vi "initImageAll.vi"() -> (3 "Refnum out":T1)   [LabVIEW 2013, in "MagAnalysis_Online.lvclass"]
uses:
  MagAnalysis_Online.lvclass
  IMAQ Image.ctl
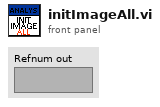
[diagram p1: front panel]
types:
  T1 = typedef "IMAQ Image.ctl" = refnum<image>
  T2 = typedef "Image Type" = u32
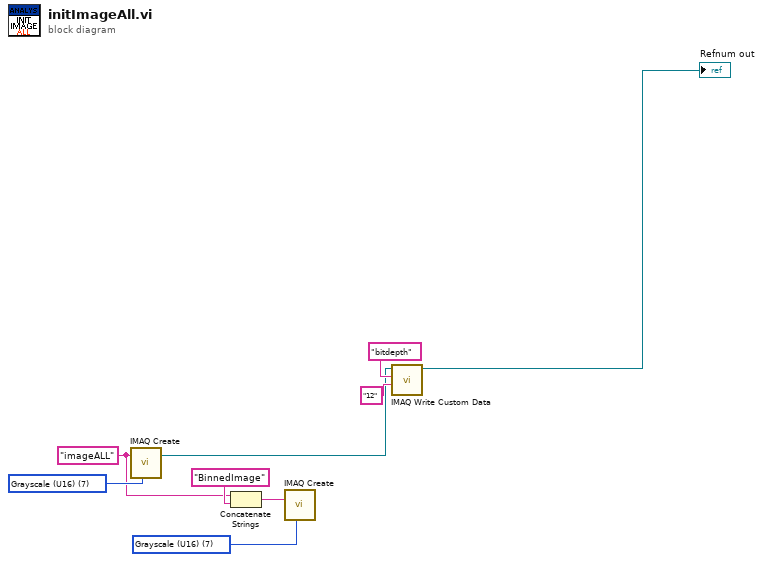
[diagram p0: block diagram]
diagram:
  w5 = T2 7 items=["Grayscale (U8)", "Grayscale (I16)", "Grayscale (SGL)", "Complex (CSG)", "RGB (U32)", "HSL (U32)", "RGB (U64)", "Grayscale (U16)"] ("Image Type")
  w9 = T2 7 items=["Grayscale (U8)", "Grayscale (I16)", "Grayscale (SGL)", "Complex (CSG)", "RGB (U32)", "HSL (U32)", "RGB (U64)", "Grayscale (U16)"] ("Image Type")
  w6 = "imageALL" ("Image Name")
  n1 = call "IMAQ Create"("Image Name"=w6, "Image Type"=w9) -> ("New Image"=w2:T1)  [unwired: 3 in, 1 out]
  n2 = Concatenate Strings(w6, "BinnedImage") -> (w8:string)
  n3 = call "IMAQ Create"("Image Name"=w8, "Image Type"=w5) -> ()  [unwired: 3 in, 2 out]
  n4 = call "IMAQ Write Custom Data"("Custom Data In"="12", "Key"="bitdepth", "Image"=w2) -> ("Image Out"=→"Refnum out":T1)  [unwired: 7 in, 1 out]
